vi "Get Columns.vi"(8 "error in":errorcluster, 10 "Sheet Name":string, 11 "SpreadsheetDoc in":refnum<k24>) -> (0 "error out":errorcluster, 2 "Columns":refnum<k24>, 3 "SpreadsheetDoc out":refnum<k24>)   [LabVIEW 2019, in "Open Xml.lvlib"]
uses:
  Open Xml.lvlib
  D:/git/Open-Xml-LabVIEW/Source/DocumentFormat.OpenXml.dll
  DocumentFormat.OpenXml.dll
  D:/git/Open-Xml-LabVIEW/Source/DocumentFormat.OpenXml.Framework.dll
  DocumentFormat.OpenXml.Framework.dll
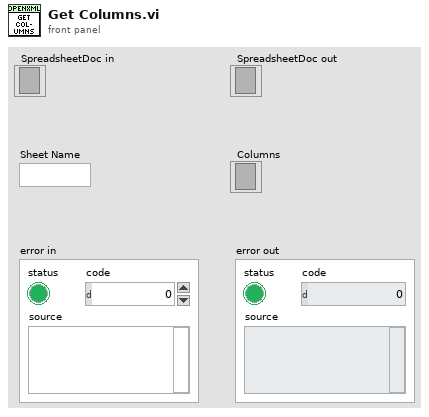
[diagram p1: front panel]
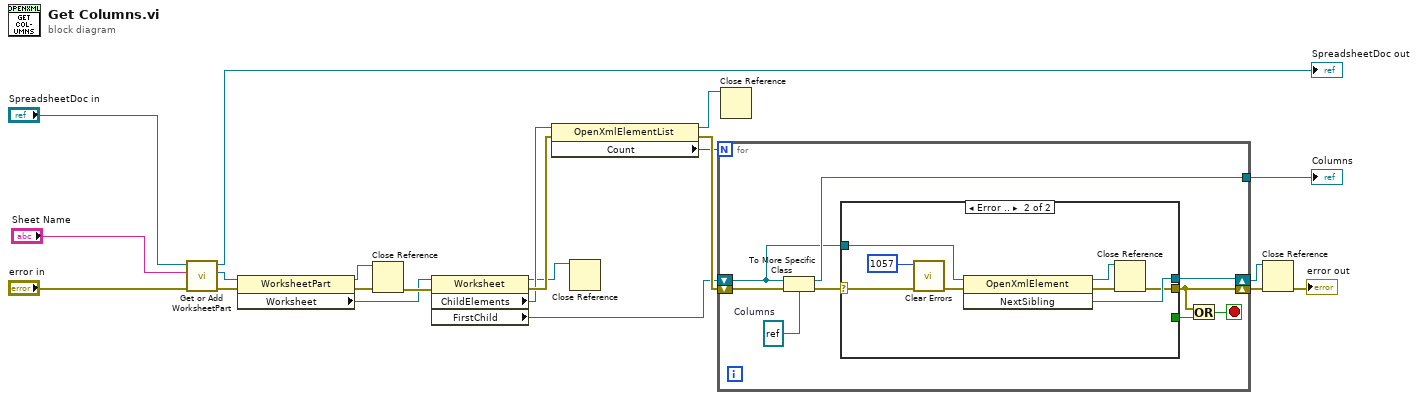
[diagram p0: block diagram]
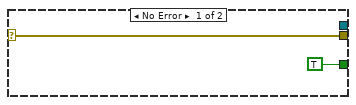
[diagram p2: hidden frame]
diagram:
  n1 = call "Get or Add WorksheetPart.vi"("error in"="error in", "Sheet Name"="Sheet Name", "SpreadsheetDoc in"="SpreadsheetDoc in") -> ("error out"=w5:errorcluster, "WorksheetPart"=w2:refnum<k24>, "SpreadsheetDoc out"=→"SpreadsheetDoc out":refnum<k24>)  [unwired: 6 in]
  n2 = property class="WorksheetPart"(reference=w2, error in=w5) -> (reference out=w8:refnum<k24>, error out=w9:errorcluster, "Worksheet"=w7:refnum<k24>)
  n3 = Close Reference(reference=w8, error in (no error)=w9) -> (error out=w10:errorcluster)
  n4 = property class="Worksheet"(reference=w7, error in=w10) -> (reference out=w1:refnum<k24>, error out=w16:errorcluster, "ChildElements"=w11:refnum<k24>, "FirstChild"=w13:refnum<k24>)
  n5 = property class="OpenXmlElementList"(reference=w11, error in=w16) -> (reference out=w15:refnum<k24>, error out=w17:errorcluster, "Count"=w14:i32)
  n6 = Close Reference(reference=w1) -> ()  [unwired: 1 in, 1 out]
  n7 = for {
    N: w14 -> [_]
    shift-right: [w24] -> w12
    shift-left: w17 -> [w30]
    shift-right: [w25] -> w20
    shift-left: w13 -> [w26]
    tunnel: [w27] -> w18
    stop <- w23 stop-if-true
    w28 = refnum<k24> refnum  # Columns
    n8 = To More Specific Class(target class=w28, reference=w26, error in=w30) -> (specific class reference=w27:refnum<k24>, error out=w29:errorcluster)
    n9 = case shown="Error .." w29 {
      selector: w29 -> [w32 w39]
      tunnel: [w32 w34] -> w24
      tunnel: w26 -> [_ w36]
      tunnel: [_ w35] -> w25
      tunnel: [TRUE _] -> w22
      frame No Error {
      }
      frame Error {
        n10 = call <vilib>:"Clear Errors.vi"("error in (no error)"=w39, "specific error code to clear (0: all)"=1057) -> ("error out"=w38:errorcluster)  [unwired: 4 in, 1 out]
        n11 = invoke class="OpenXmlElement" method="NextSibling"(reference=w36, error in=w38) -> (reference out=w33:refnum<k24>, error out=w40:errorcluster, "NextSibling"=w35:refnum<k24>)  [unwired: 1 in]
        n12 = Close Reference(reference=w33, error in (no error)=w40) -> (error out=w34:errorcluster)
      }
    }
    n13 = Or(x=w24, y=w22) -> (x .or. y?=w23:bool)
  }
  "Columns" <- w18
  n14 = Close Reference(reference=w15) -> ()  [unwired: 1 in, 1 out]
  n15 = Close Reference(reference=w20, error in (no error)=w12) -> (error out=→"error out":errorcluster)
